vi "ExecLog_LogLabViewError.vi"(0 "error IO":errorcluster, 1 "string 2":string, 2 "string 1":string) -> ()   [LabVIEW 2017]
uses:
  <vilib>/Utility/error.llb/DialogType.ctl
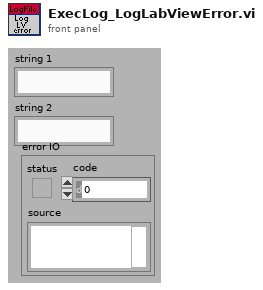
[diagram p1: front panel]
types:
  T1 = typedef "DialogType.ctl" = u16
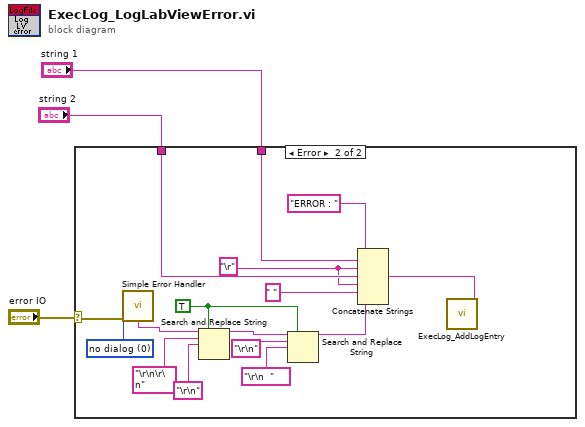
[diagram p0: block diagram]
diagram:
  n1 = case shown="Error" "error IO" {
    selector: "error IO" -> [_ w19]
    tunnel: "string 2" -> [_ w16]
    tunnel: "string 1" -> [_ w7]
    frame No Error {
    }
    frame Error {
      w18 = T1 0 items=["no dialog", "OK message", "continue or stop message", "OK message + warnings", "continue/stop + warnings"] ("type of dialog (OK msg:1)")
      w4 = "\r" ("search string")
      w14 = TRUE ("replace all? (F)")
      n2 = call <vilib>:"Simple Error Handler.vi"("type of dialog (OK msg:1)"=w18, "error in (no error)"=w19) -> ("message"=w15:string)  [unwired: 7 out]
      n3 = Search and Replace String(replace all?=w14, input string=w15, search string="\r\n\r\n", replace string="\r\n" ("search string")) -> (result string=w13:string)  [unwired: 1 in, 6 out]
      n4 = Search and Replace String(replace all?=w14, input string=w13, search string="\r\n", replace string="\r\n  " ("replace string (\"\")")) -> (result string=w8:string)  [unwired: 1 in, 6 out]
      n5 = Concatenate Strings("ERROR : " ("string"), w7, w4, w16, w4, " " ("string"), w8) -> (w17:string)
      n6 = call "ExecLog_AddLogEntry.vi"("Msg"=w17) -> ()  [unwired: 8 in, 3 out]
    }
  }
